vi "tsflexray_set_controller_frametrigger.vi"() -> ()   [LabVIEW 2014]
doc: "TSAPI(s32)tsflexray_set_controller_frametrigger(const s32 AIdxChn,const PLIBFlexray_controller_config AControllerConfig,const ps32 AFrameLengthArray,const s32 AFrameNum,const PLIBTrigger_def AFrameTrigger,const s32 AFrameTriggerNum,const s32 ATimeoutMs);"
panel:
  out "path out":path
  in  "path in":path
  out "error out":errorcluster caption="错误输出"
  in  "error in (no error)":errorcluster caption="错误输入（无错误）"
  in  "ATimeoutMs":i32
  in  "AFrameTriggerNum":i32
  in  "AFrameTrigger":T1
  in  "AFrameNum":i32
  in  "AFrameLengthArray":i32
  in  "AControllerConfig":T2
  in  "AIdxChn":i32
  out "function return":i32
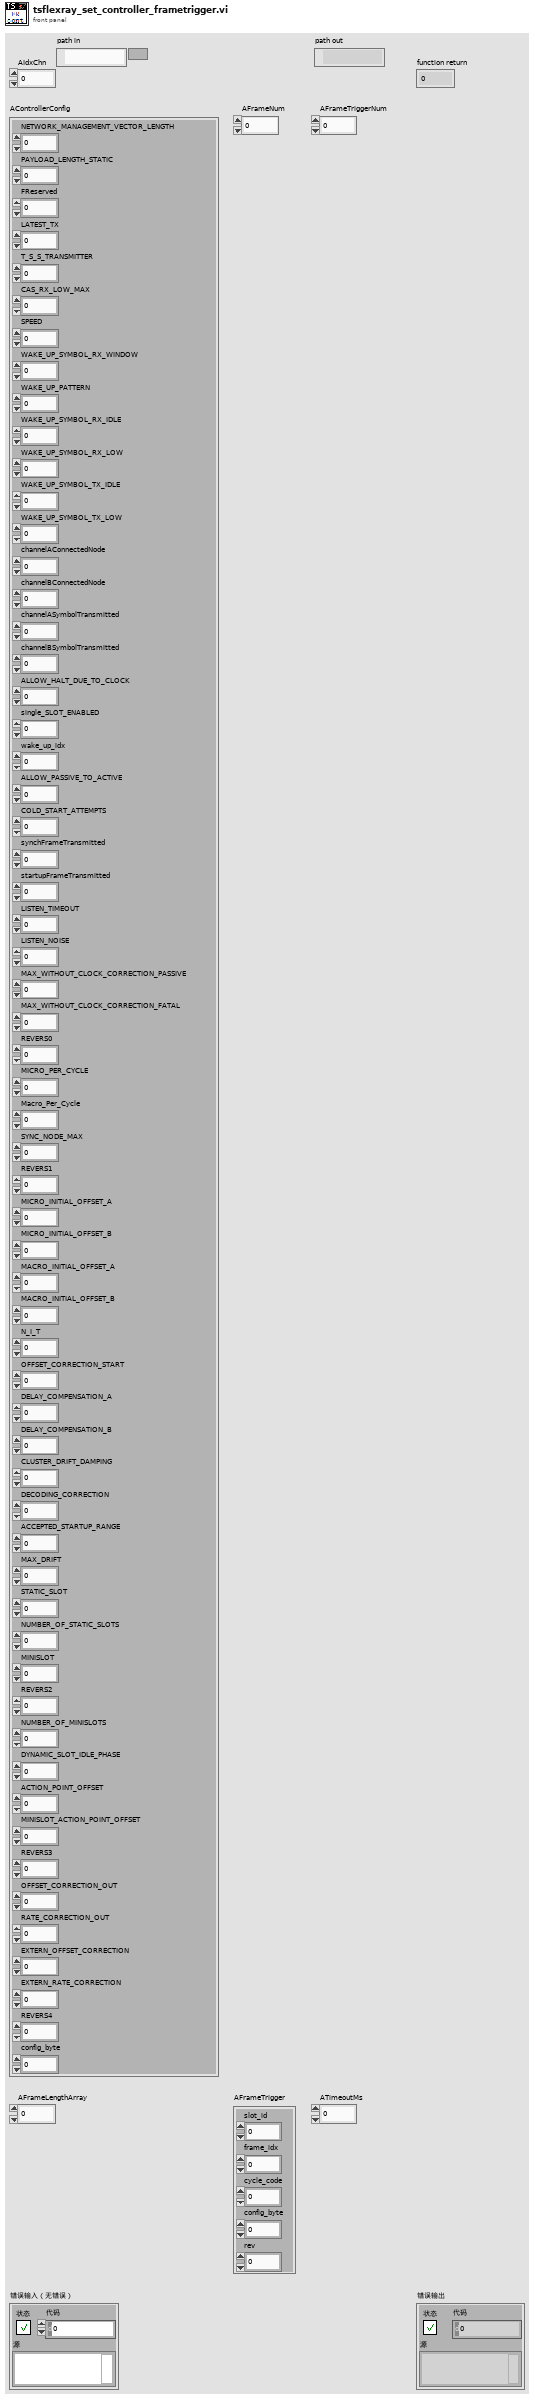
[diagram p1: front panel]
types:
  T1 = cluster{"slot_id":u32, "frame_idx":u8, "cycle_code":u8, "config_byte":u8, "rev":u8}
  T2 = cluster{"NETWORK_MANAGEMENT_VECTOR_LENGTH":u8, "PAYLOAD_LENGTH_STATIC":u8, "FReserved":u32, "LATEST_TX":u32, "T_S_S_TRANSMITTER":u32, "CAS_RX_LOW_MAX":u8, "SPEED":u8, "WAKE_UP_SYMBOL_RX_WINDOW":u32, "WAKE_UP_PATTERN":u8, "WAKE_UP_SYMBOL_RX_IDLE":u8, "WAKE_UP_SYMBOL_RX_LOW":u8, "WAKE_UP_SYMBOL_TX_IDLE":u8, "WAKE_UP_SYMBOL_TX_LOW":u8, "channelAConnectedNode":u8, "channelBConnectedNode":u8, "channelASymbolTransmitted":u8, "channelBSymbolTransmitted":u8, "ALLOW_HALT_DUE_TO_CLOCK":u8, "single_SLOT_ENABLED":u8, "wake_up_idx":u8, "ALLOW_PASSIVE_TO_ACTIVE":u8, "COLD_START_ATTEMPTS":u8, "synchFrameTransmitted":u8, "startupFrameTransmitted":u8, "LISTEN_TIMEOUT":u32, "LISTEN_NOISE":u8, "MAX_WITHOUT_CLOCK_CORRECTION_PASSIVE":u8, "MAX_WITHOUT_CLOCK_CORRECTION_FATAL":u8, "REVERS0":u8, "MICRO_PER_CYCLE":u32, "Macro_Per_Cycle":u32, "SYNC_NODE_MAX":u8, "REVERS1":u8, "MICRO_INITIAL_OFFSET_A":u8, "MICRO_INITIAL_OFFSET_B":u8, "MACRO_INITIAL_OFFSET_A":u8, "MACRO_INITIAL_OFFSET_B":u8, "N_I_T":u32, "OFFSET_CORRECTION_START":u32, "DELAY_COMPENSATION_A":u8, "DELAY_COMPENSATION_B":u8, "CLUSTER_DRIFT_DAMPING":u8, "DECODING_CORRECTION":u8, "ACCEPTED_STARTUP_RANGE":u32, "MAX_DRIFT":u32, "STATIC_SLOT":u32, "NUMBER_OF_STATIC_SLOTS":u32, "MINISLOT":u8, "REVERS2":u8, "NUMBER_OF_MINISLOTS":u32, "DYNAMIC_SLOT_IDLE_PHASE":u8, "ACTION_POINT_OFFSET":u8, "MINISLOT_ACTION_POINT_OFFSET":u8, "REVERS3":u8, "OFFSET_CORRECTION_OUT":u32, "RATE_CORRECTION_OUT":u32, "EXTERN_OFFSET_CORRECTION":u8, "EXTERN_RATE_CORRECTION":u8, "REVERS4":u8, "config_byte":u8}
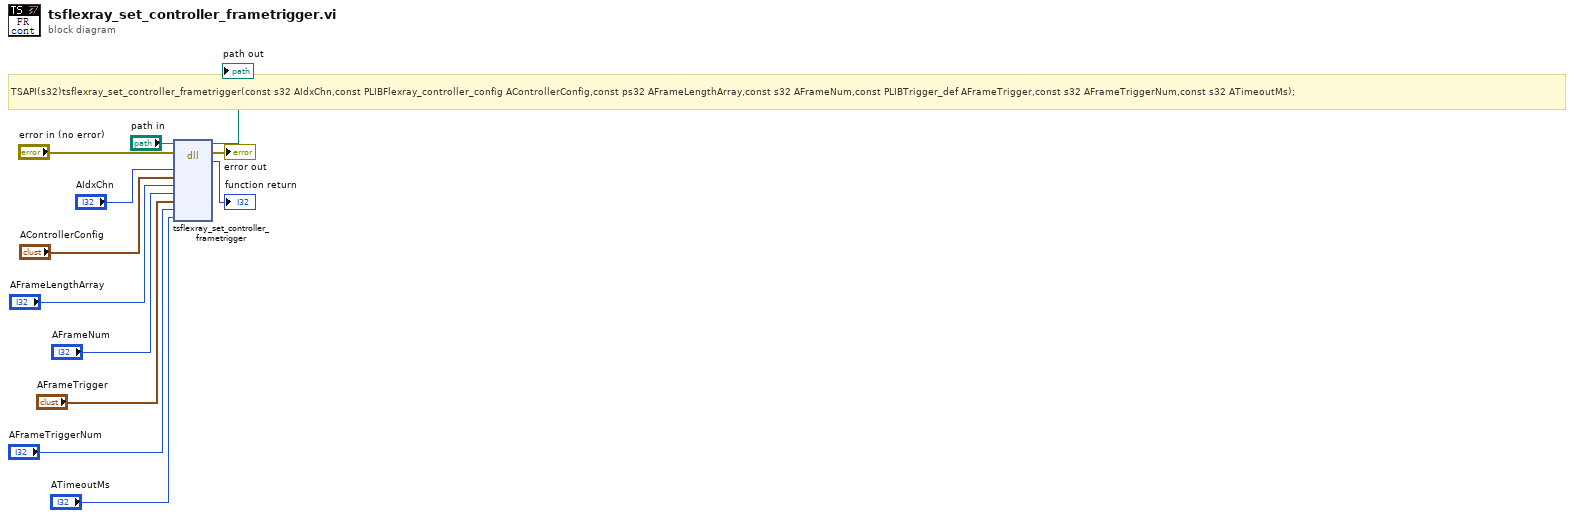
[diagram p0: block diagram]
diagram:
  # "TSAPI(s32)tsflexray_set_controller_frametrigger(const s32 AIdxChn,const PLIBFlexray_controller_config AControllerConfig,const ps32 AFrameLengthArray,const s32 AFrameNum,const PLIBTrigger_def AFrameTrigger,const s32 AFrameTriggerNum,const s32 ATimeoutMs);"
  n1 = dll-call lib="D:/Work/LabVIEW Code/TSMaster Labview SDK/LabVIEW/LabVIEW-TSMasterAPI_CLN/TSMasterAPI_LabVIEW-2024-10-08 14-20-13/Not_organized_vi/TSMaster.*" fn="tsflexray_set_controller_frametrigger"(path in="path in", error in="error in (no error)", "AIdxChn"="AIdxChn", "AControllerConfig"="AControllerConfig", "AFrameLengthArray"="AFrameLengthArray", "AFrameNum"="AFrameNum", "AFrameTrigger"="AFrameTrigger", "AFrameTriggerNum"="AFrameTriggerNum", "ATimeoutMs"="ATimeoutMs") -> (path out=→"path out":path, error out=→"error out":errorcluster, "返回类型"=→"function return":i32)  [unwired: 8 in]
